vi "Control Sys_Main.vi"(8 "error in":errorcluster, 11 "QRD":T1) -> (0 "error out":errorcluster)   [LabVIEW 2025]
uses:
  Controls/Queues-Refs-Data.ctl
  Builds/Queue Wrappers.lvlibp/Q Packet.ctl
  Controls/Local Data_Acquisition.ctl
  Controls/Acquisition Packet.ctl
  Builds/Queue Wrappers.lvlibp
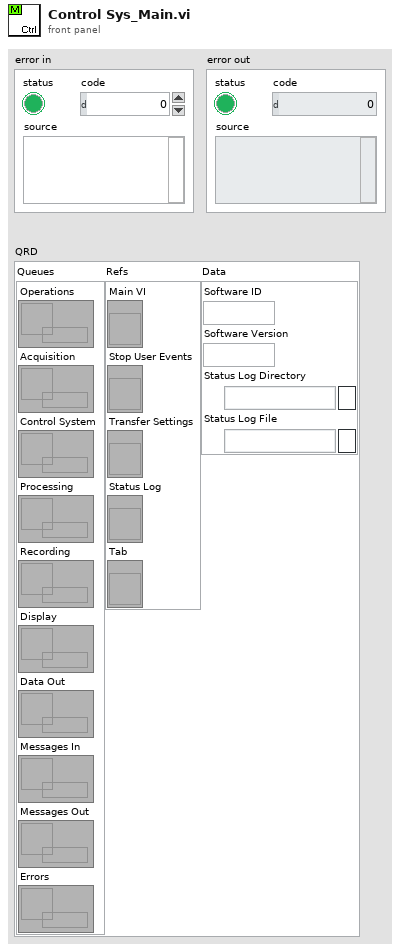
[diagram p1: front panel]
types:
  T1 = typedef "Queues-Refs-Data.ctl" = cluster{"Queues":cluster{"Operations":refnum<queue>, "Acquisition":refnum<queue>, "Control System":refnum<queue>, "Processing":refnum<queue>, "Recording":refnum<queue>, "Display":refnum<queue>, "Data Out":refnum<queue>, "Messages In":refnum<queue>, "Messages Out":refnum<queue>, "Errors":refnum<queue>}, "Refs":cluster{"Main VI":refnum<vi>, "Stop User Events":refnum<vi>, "Transfer Settings":refnum<vi>, "Status Log":refnum<vi>, "Tab":refnum<vi>}, "Data":cluster{"Software ID":string, "Software Version":string, "Status Log Directory":path, "Status Log File":path}}
  T2 = typedef "Local Data_Acquisition.ctl" = cluster{"Loop ID":string, "Transmit Interval":u32, "Last Transmit":timestamp}
  T3 = typedef "Acquisition Packet.ctl" = cluster{"Time Stamp":timestamp, "Raw Data":cluster{"String":string, "Numeric":dbl, "Boolean":bool}, "Derived Data":cluster{"String":string, "Numeric":dbl, "Boolean":bool}}
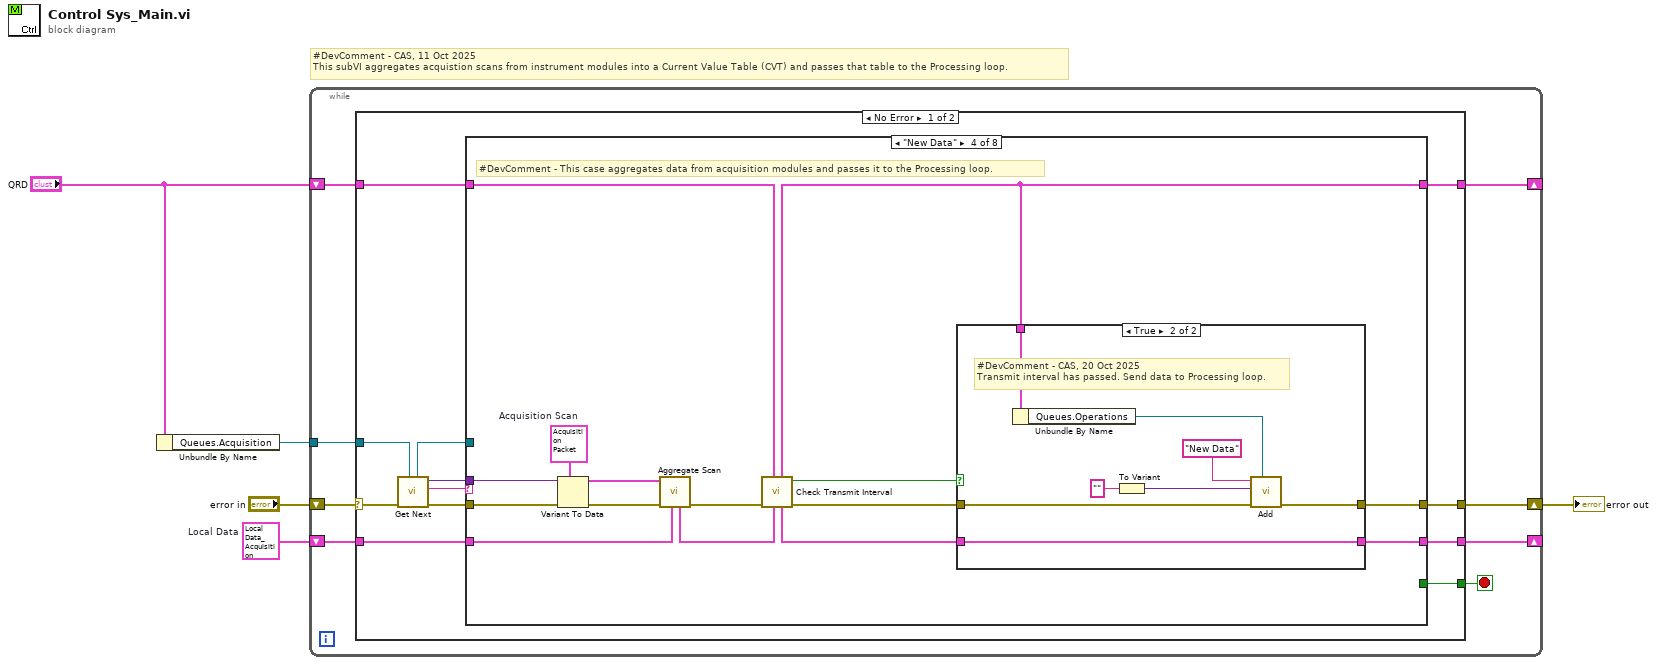
[diagram p0: block diagram]
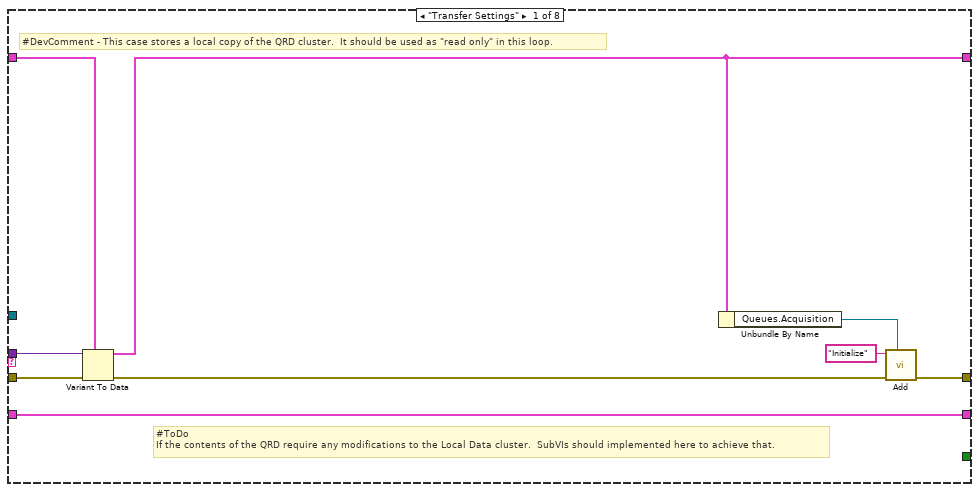
[diagram p2: hidden frame]
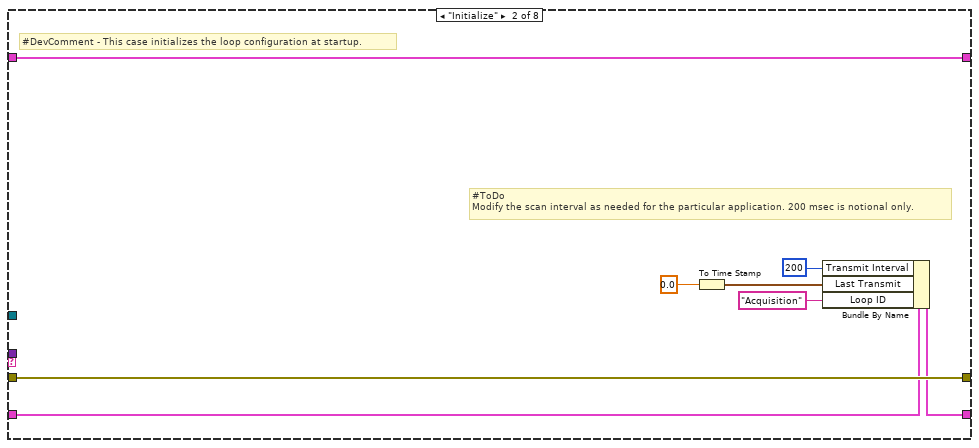
[diagram p3: hidden frame]
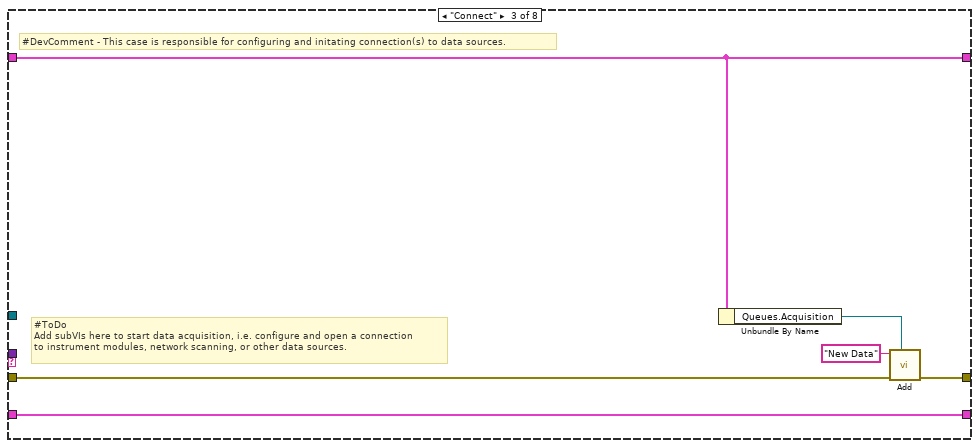
[diagram p4: hidden frame]
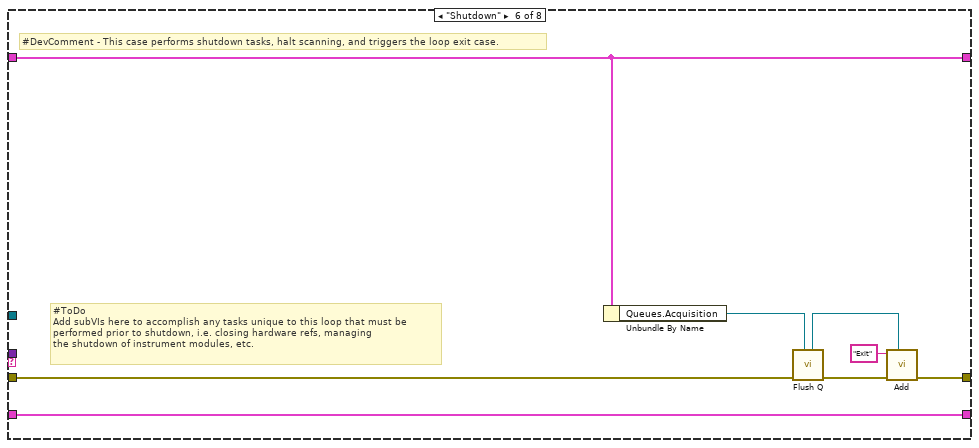
[diagram p7: hidden frame]
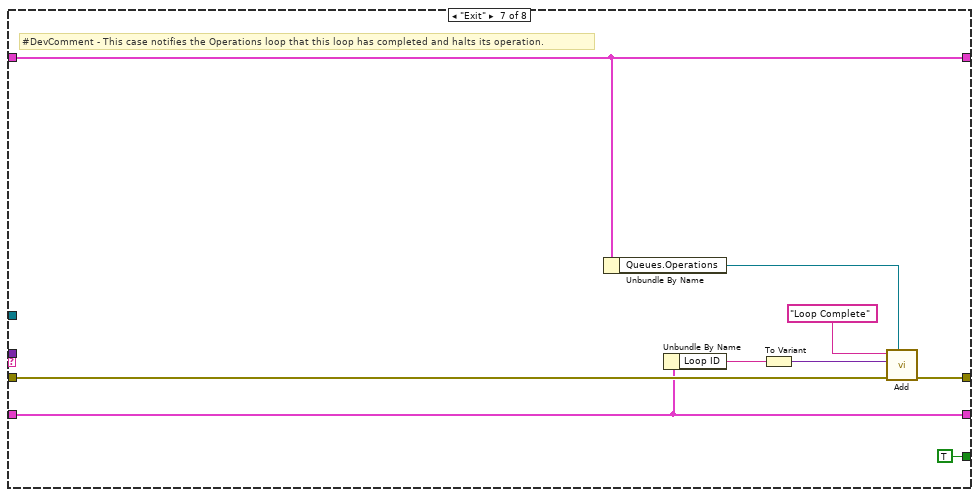
[diagram p8: hidden frame]
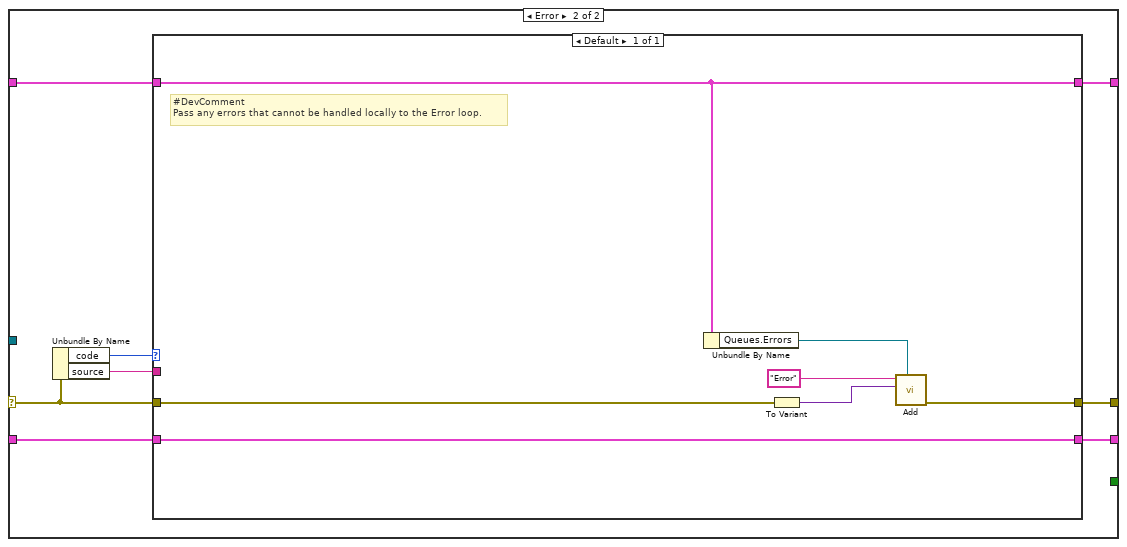
[diagram p10: hidden frame]
diagram:
  w3 = T2 {"Loop ID"="", "Transmit Interval"=0, "Last Transmit"=timestamp(0 s since 1904-01-01)}  # Local Data
  # "#DevComment - CAS, 11 Oct 2025\nThis subVI aggregates acquistion scans from instrument modules into a Current Value Table (CVT) and passes that table to the Processing loop."
  n1 = Unbundle By Name("QRD") -> ("Queues.Acquisition"=w1:refnum<queue>)
  n2 = while {
    shift-right: [w12] -> _
    shift-left: "QRD" -> [w13]
    shift-right: [w10] -> w5
    shift-left: "error in" -> [w11]
    tunnel: w1 -> [w9]
    shift-right: [w7] -> _
    shift-left: w3 -> [w8]
    stop <- w6 stop-if-true
    n3 = case shown="No Error" w11 {
      selector: w11 -> [w25 w100]
      tunnel: w13 -> [w22 w97]
      tunnel: [w23 w98] -> w12
      tunnel: [w20 w99] -> w10
      tunnel: w9 -> [w24 _]
      tunnel: w8 -> [w16 w102]
      tunnel: [w15 w101] -> w7
      tunnel: [w14 _] -> w6
      frame No Error {
        n4 = call "Get Next.vi"("Q Ref In"=w24, "error in"=w25) -> ("error out"=w21:errorcluster, "Packet ID"=w17:string, "Payload"=w18:variant, "Q Ref Out"=w19:refnum<queue>)  [unwired: 6 in]
        n5 = case shown="\"New Data\"" w17 {
          tunnel: [w28 w42 w46 w50 w74 w84 w93 w96] -> w23
          tunnel: w22 -> [w31 w42 w46 w55 w74 w84 w93 w96]
          tunnel: w21 -> [w33 w41 w47 w63 w76 w80 w90 w95]
          tunnel: [w29 w41 w44 w53 w76 w82 w92 w95] -> w20
          tunnel: w19 -> [_ _ _ _ _ _ _ _]
          tunnel: w18 -> [w32 _ _ w62 _ _ _ _]
          tunnel: w16 -> [w34 w40 w48 w58 w75 w83 w88 w94]
          tunnel: [w34 w39 w48 w52 w75 w83 w88 w94] -> w15
          tunnel: [_ _ _ _ _ _ TRUE _] -> w14
          frame "Transfer Settings" {
            # "#ToDo\nIf the contents of the QRD require any modifications to the Local Data cluster.  SubVIs should implemented here to achieve that."
            # "#DevComment - This case stores a local copy of the QRD cluster.  It should be used as \"read only\" in this loop."
            n6 = Variant To Data(error in=w33, type=w31, Variant=w32) -> (data=w28:T1, error out=w30:errorcluster)
            n7 = Unbundle By Name(w28) -> ("Queues.Acquisition"=w27:refnum<queue>)
            n8 = call "Add.vi"("Q Ref In"=w27, "error in"=w30, "Packet ID"="Initialize") -> ("error out"=w29:errorcluster)  [unwired: 5 in, 3 out]
          }
          frame "Initialize" {
            # "#ToDo\nModify the scan interval as needed for the particular application. 200 msec is notional only."
            # "#DevComment - This case initializes the loop configuration at startup."
            n9 = To Time Stamp(1:0.0) -> (0:w35:timestamp)
            n10 = Bundle By Name(cluster=w40, "Transmit Interval"=u32 200 ("Scan Interval"), "Last Transmit"=w35, "Loop ID"="Acquisition") -> (w39:T2)
          }
          frame "Connect" {
            # "#ToDo\nAdd subVIs here to start data acquisition, i.e. configure and open a connection\nto instrument modules, network scanning, or other data sources."
            # "#DevComment - This case is responsible for configuring and initating connection(s) to data sources."
            n11 = Unbundle By Name(w46) -> ("Queues.Acquisition"=w45:refnum<queue>)
            n12 = call "Add.vi"("Q Ref In"=w45, "error in"=w47, "Packet ID"="New Data") -> ("error out"=w44:errorcluster)  [unwired: 5 in, 3 out]
          }
          frame "New Data" {
            w61 = T3 {"Time Stamp"=timestamp(0 s since 1904-01-01), "Raw Data"={"String"="", "Numeric"=0.0, "Boolean"=FALSE}, "Derived Data"={"String"="", "Numeric"=0.0, "Boolean"=FALSE}}  # Acquisition Scan
            # "#DevComment - This case aggregates data from acquisition modules and passes it to the Processing loop."
            n13 = Variant To Data(error in=w63, type=w61, Variant=w62) -> (data=w59:T3, error out=w60:errorcluster)
            n14 = call "Aggregate Scan.vi"("Local Data"=w58, "error in"=w60, "Acquisition Scan"=w59) -> ("error out"=w57:errorcluster, "Local Data Out"=w56:T2)  [unwired: 7 in]
            n15 = call "Check Transmit Interval.vi"("Local Data"=w56, "QRD"=w55, "error in"=w57) -> ("error out"=w54:errorcluster, "Transmit Data?"=w49:bool, "Local Data Out"=w51:T2, "QRD Out"=w50:T1)  [unwired: 5 in]
            n16 = case shown="True" w49 {
              tunnel: w50 -> [_ w73]
              tunnel: w54 -> [w65 w71]
              tunnel: [w65 w70] -> w53
              tunnel: w51 -> [w64 w67]
              tunnel: [w64 w67] -> w52
              frame False {
                # "#DevComment - CAS, 20 Oct 2025\nTransmit interval has not passed."
              }
              frame True {
                # "#DevComment - CAS, 20 Oct 2025\nTransmit interval has passed. Send data to Processing loop."
                n17 = Unbundle By Name(w73) -> ("Queues.Operations"=w72:refnum<queue>)
                n18 = To Variant(anything="") -> (Variant=w68:variant)
                n19 = call "Add.vi"("Q Ref In"=w72, "error in"=w71, "Payload"=w68, "Packet ID"="New Data") -> ("error out"=w70:errorcluster)  [unwired: 4 in, 3 out]
              }
            }
          }
          frame "Disconnect" {
            # "#ToDo"
            # "#DevComment - This case commands the shutdown of acquisition modules."
          }
          frame "Shutdown" {
            # "#ToDo\nAdd subVIs here to accomplish any tasks unique to this loop that must be\nperformed prior to shutdown, i.e. closing hardware refs, managing\nthe shutdown of instrument modules, etc."
            # "#DevComment - This case performs shutdown tasks, halt scanning, and triggers the loop exit case."
            n20 = Unbundle By Name(w84) -> ("Queues.Acquisition"=w78:refnum<queue>)
            n21 = call "Flush Q.vi"("Q Ref In"=w78, "error in"=w80) -> ("error out"=w79:errorcluster, "Q Ref Out"=w77:refnum<queue>)  [unwired: 8 in]
            n22 = call "Add.vi"("Q Ref In"=w77, "error in"=w79, "Packet ID"="Exit") -> ("error out"=w82:errorcluster)  [unwired: 5 in, 3 out]
          }
          frame "Exit" {
            # "#DevComment - This case notifies the Operations loop that this loop has completed and halts its operation."
            n23 = Unbundle By Name(w93) -> ("Queues.Operations"=w89:refnum<queue>)
            n24 = Unbundle By Name(w88) -> ("Loop ID"=w87:string)
            n25 = To Variant(anything=w87) -> (Variant=w86:variant)
            n26 = call "Add.vi"("Q Ref In"=w89, "error in"=w90, "Payload"=w86, "Packet ID"="Loop Complete") -> ("error out"=w92:errorcluster)  [unwired: 4 in, 3 out]
          }
          frame Default {
          }
        }
      }
      frame Error {
        n27 = Unbundle By Name(w100) -> ("code"=w104:i32, "source"=w103:string)
        n28 = case shown="Default" w104 {
          tunnel: w103 -> [_]
          tunnel: w102 -> [w111]
          tunnel: [w111] -> w101
          tunnel: w100 -> [w106]
          tunnel: [w108] -> w99
          tunnel: [w107] -> w98
          tunnel: w97 -> [w107]
          frame Default {
            # "#DevComment\nPass any errors that cannot be handled locally to the Error loop."
            n29 = Unbundle By Name(w107) -> ("Queues.Errors"=w109:refnum<queue>)
            n30 = To Variant(anything=w106) -> (Variant=w105:variant)
            n31 = call "Add.vi"("Q Ref In"=w109, "Payload"=w105, "Packet ID"="Error") -> ("error out"=w108:errorcluster)  [unwired: 5 in, 3 out]
          }
        }
      }
    }
  }
  "error out" <- w5
